vi "format_tpg361_data.vi"(10 "pressure":dbl, 11 "time":timestamp) -> (2 "pressure_out":dbl, 3 "waveform_array":waveform(dbl)[](array[waveform]))   [LabVIEW 2019]
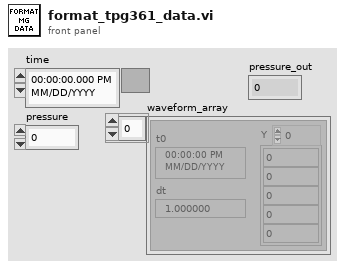
[diagram p1: front panel]
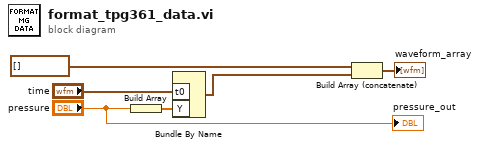
[diagram p0: block diagram]
diagram:
  n1 = Build Array("pressure") -> (w5:dbl[])
  n2 = Bundle By Name("t0"="time", "Y"=w5) -> (w4:waveform(dbl))  [unwired: 1 in]
  n3 = Build Array (concatenate)(waveform(dbl)[] [], w4) -> (→"waveform_array":waveform(dbl)[])
  "pressure_out" <- "pressure"
